vi "Param_Analysis_7_24a_JW.vi"(7 "error in (no error)":errorcluster, 8 "Data Folder":path=path "D:/Userdata/Documents/Lab/8_26/diF-TES ADT 0_33pct cB_SAC-Shaker/data", 9 "Parameter String":string, 10 "Parameter Name":string, 11 "Stats Folder":path=path "D:/Userdata/Documents/Lab/8_26/diF-TES ADT 0_33pct cB_SAC-Shaker/data") -> (0 "Output File":path=path "D:/Userdata/Documents/Lab/8_26/diF-TES ADT 0_33pct cB_SAC-Shaker/data", 1 "error out":errorcluster, 2 "Histogram Array":string[](array[string]), 3 "Param vs L Array":string[][](array[string]))   [LabVIEW 2011]
doc: "Stats Folder - Directory where the analysis is to be stored\n\nData Folder - Directory where the files to be analyzed are stored\n\nParameter Name - String to be used as the name of the outputed file for the analyzed paramters \n\nParameter String - String that should be identically equal to the name adjacent to the parameter to be analyzed in the data files\n\n\nOutput File - Directory where the analysis summary is located"
uses:
  <vilib>/Utility/file.llb/Write To Spreadsheet File (string).vi
  <vilib>/Utility/file.llb/Read From Spreadsheet File (string).vi
panel:
  out "Output Array":string[][](array[string])
  out "Parameter String 2":string
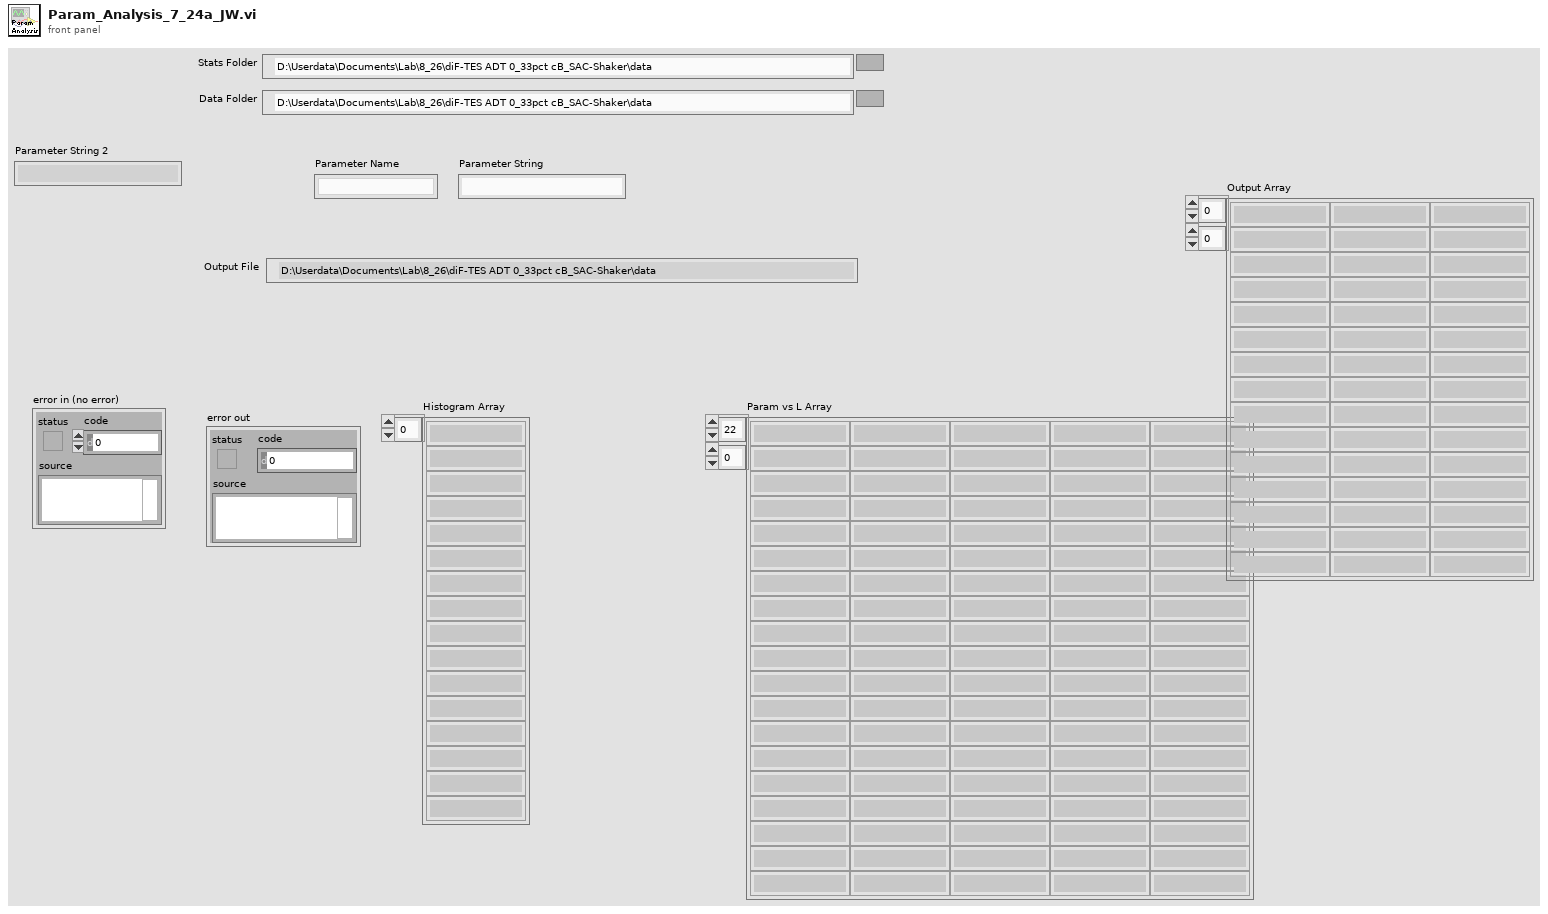
[diagram p1: front panel]
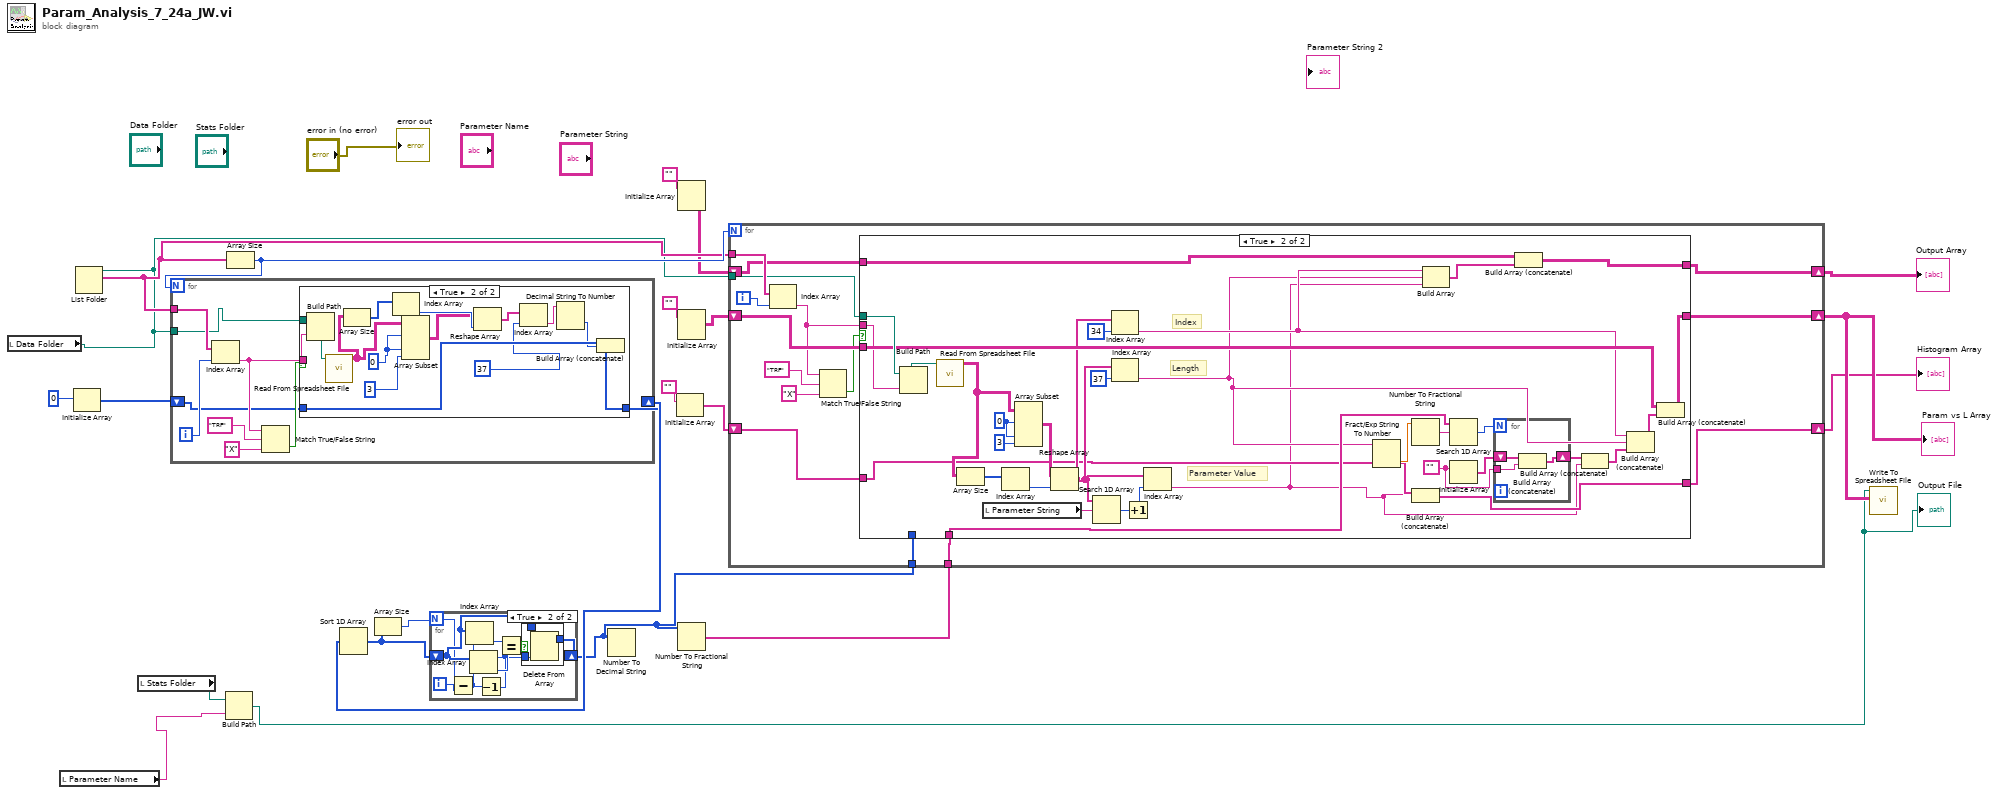
[diagram p0: block diagram]
diagram:
  n1 = local read "Data Folder"() -> (w7:path)
  n2 = local read "Parameter Name"() -> (w6:string)
  n3 = Initialize Array(0) -> (w16:i32[])  [unwired: 1 in]
  n4 = List Folder(path=w7) -> (filenames=w22:string[])  [unwired: 3 in, 3 out]
  n5 = local read "Stats Folder"() -> (w13:path)
  n6 = Build Path(base path=w13, name or relative path=w6) -> (appended path=w5:path)
  "Output File" <- w5
  n7 = Array Size(array=w22) -> (size(s)=w23:i32)
  n8 = for {
    N: w23 -> [_]
    tunnel: w22 -> [w32]
    tunnel: w7 -> [w30]
    shift-right: [w25] -> w21
    shift-left: w16 -> [w24]
    i -> [w31]
    n9 = Index Array(array=w32, index=w31) -> (element=w29:string)
    n10 = Match True/False String(2:"X", 3:"TRF", 4:w29) -> (0:w27:bool)  [unwired: 1 out]
    n11 = case shown="True" w27 {
      tunnel: w30 -> [_ w48]
      tunnel: w29 -> [_ w40]
      tunnel: [w33 w39] -> w25
      tunnel: w24 -> [w33 w38]
      frame False {
      }
      frame True {
        w45 = 0
        n12 = Build Path(base path=w48, name or relative path=w40) -> (appended path=w47:path)
        n13 = call-poly <vilib>:"Read From Spreadsheet File.vi"("file path (dialog if empty)"=w47) -> ("all rows"=w43:string[][])  [unwired: 6 in, 4 out]
        n14 = Array Size(array=w43) -> (size(s)=w44:i32[])
        n15 = Index Array(array=w44) -> (element=w42:i32)  [unwired: 1 in]
        n16 = Array Subset(array=w43, index (row)=w45, index (col)=w45, length (col)=3) -> (w41:string[][])  [unwired: 1 in]
        n17 = Reshape Array(w41, w42) -> (w35:string[])
        n18 = Index Array(array=w35, index=37) -> (element=w37:string)
        n19 = Decimal String To Number(string=w37) -> (number=w36:i32)  [unwired: 2 in, 1 out]
        n20 = Build Array (concatenate)(w38, w36) -> (w39:i32[])
      }
    }
  }
  n21 = Sort 1D Array(array=w21) -> (sorted array=w20:i32[])
  n22 = Array Size(array=w20) -> (size(s)=w19:i32)
  n23 = for {
    N: w19 -> [w52]
    shift-right: [w49] -> w11
    shift-left: w20 -> [w54]
    i -> [w53]
    n24 = Subtract(x=w52, y=w53) -> (x-y=w51:i32)
    n25 = Index Array(array=w54, index=w51) -> (element=w56:i32)
    n26 = Decrement(x=w51) -> (x-1=w50:i32)
    n27 = Index Array(array=w54, index=w50) -> (element=w57:i32)
    n28 = Equal?(x=w56, y=w57) -> (x = y?=w55:bool)
    n29 = case shown="True" w55 {
      tunnel: w54 -> [w58 w61]
      tunnel: w50 -> [_ w60]
      tunnel: [w58 w59] -> w49
      frame False {
      }
      frame True {
        n30 = Delete From Array(array=w61, index=w60) -> (array with subset deleted=w59:i32[])  [unwired: 1 in, 1 out]
      }
    }
  }
  n31 = Number To Decimal String(number=w11) -> ()  [unwired: 1 in, 1 out]
  n32 = Initialize Array("") -> (w3:string[])  [unwired: 1 in]
  n33 = Initialize Array("") -> (w1:string[][])  [unwired: 2 in]
  n34 = Initialize Array("") -> (w10:string[][])  [unwired: 2 in]
  n35 = Number To Fractional String(number=w11) -> (F-format string=w14:string[])  [unwired: 3 in]
  n36 = for {
    N: w23 -> [_]
    tunnel: w22 -> [w76]
    tunnel: w7 -> [w74]
    shift-right: [w72] -> w15
    shift-left: w10 -> [w73]
    tunnel: w14 -> [w67]
    tunnel: w11 -> [w66]
    shift-right: [w64] -> w8
    shift-left: w3 -> [w65]
    shift-right: [w63] -> w4
    shift-left: w1 -> [w62]
    i -> [w75]
    n37 = Index Array(array=w76, index=w75) -> (element=w71:string)
    n38 = Match True/False String(2:"X", 3:"TRF", 4:w71) -> (0:w69:bool)  [unwired: 1 out]
    n39 = case shown="True" w69 {
      tunnel: w74 -> [_ w113]
      tunnel: w73 -> [w79 w103]
      tunnel: [w79 w101] -> w72
      tunnel: w71 -> [_ w100]
      tunnel: w67 -> [_ w89]
      tunnel: w66 -> [_ _]
      tunnel: w65 -> [w78 w87]
      tunnel: [w78 w88] -> w64
      tunnel: [w77 w81] -> w63
      tunnel: w62 -> [w77 w80]
      frame False {
      }
      frame True {
        w96 = ""
        w110 = 0
        # "Parameter Value"
        # "Length"
        # "Index"
        n40 = Build Path(base path=w113, name or relative path=w100) -> (appended path=w112:path)
        n41 = call-poly <vilib>:"Read From Spreadsheet File.vi"("file path (dialog if empty)"=w112) -> ("all rows"=w108:string[][])  [unwired: 6 in, 4 out]
        n42 = Array Size(array=w108) -> (size(s)=w109:i32[])
        n43 = local read "Parameter String"() -> (w86:string)
        n44 = Index Array(array=w109) -> (element=w107:i32)  [unwired: 1 in]
        n45 = Array Subset(array=w108, index (row)=w110, index (col)=w110, length (col)=3) -> (w106:string[][])  [unwired: 1 in]
        n46 = Reshape Array(w106, w107) -> (w93:string[])
        n47 = Search 1D Array(1D array=w93, element=w86) -> (index of element=w94:i32)  [unwired: 1 in]
        n48 = Index Array(array=w93, index=34) -> (element=w85:string)
        n49 = Index Array(array=w93, index=37) -> (element=w84:string)
        n50 = Increment(x=w94) -> (x+1=w92:i32)
        n51 = Index Array(array=w93, index=w92) -> (element=w83:string)
        n52 = Fract/Exp String To Number(string=w84) -> (number=w91:dbl)  [unwired: 3 in, 1 out]
        n53 = Number To Fractional String(number=w91) -> (F-format string=w90:string)  [unwired: 3 in]
        n54 = Build Array (concatenate)(w87, w83) -> (w88:string[])
        n55 = Build Array(w85, w84, w83) -> (w82:string[])
        n56 = Search 1D Array(1D array=w89, element=w90) -> (index of element=w95:i32)  [unwired: 1 in]
        n57 = Initialize Array(w96) -> (w97:string[])  [unwired: 1 in]
        n58 = for {
          N: w95 -> [_]
          shift-right: [w115] -> w99
          shift-left: w97 -> [w116]
          tunnel: w96 -> [w114]
          n59 = Build Array (concatenate)(w116, w114) -> (w115:string[])
        }
        n60 = Build Array (concatenate)(w80, w82) -> (w81:string[][])
        n61 = Build Array (concatenate)(w99, w83) -> (w98:string[])
        n62 = Build Array (concatenate)(w85, w84, w98) -> (w102:string[])
        n63 = Build Array (concatenate)(w103, w102) -> (w101:string[][])
      }
    }
  }
  "Param vs L Array" <- w15
  "Histogram Array" <- w8
  "Output Array" <- w4
  n64 = call-poly <vilib>:"Write To Spreadsheet File.vi"("2D data"=w15, "file path (dialog if empty)"=w5) -> ()  [unwired: 6 in, 1 out]
  "error out" <- "error in (no error)"
